vi "NI VeriStand - Start Multiple Waveforms Multi t0 (DBL).vi"(8 "error in (no error)":errorcluster, 10 "t0s":timestamp[](array[timestamp]), 11 "Multiple Waveforms Write Session (DBL) in":refnum<class "Multiple Waveforms Write (DBL).lvclass">) -> (0 "error out":errorcluster, 3 "Multiple Waveforms Write Session (DBL) out":refnum<class "Multiple Waveforms Write (DBL).lvclass">)   [LabVIEW 2020, in "NI_VS Custom Device Waveform API.lvlib" / "Multiple Waveforms Write (DBL).lvclass"]
doc: "Sets the start time (t0) for the waveform data you want to write with the Write Waveform(s) VI. NI VeriStand considers all data the custom device writes to a waveform be continuous unless this VI executes again with a different start time."
uses:
  Multiple Waveforms Write (DBL).lvclass
  D:/p4/penguin/lvaddon/Veristand/master/src/LabVIEW/vilib/NI VeriStand/Custom Device Waveform API/Waveform Session.lvclass
  Waveform Session.lvclass/Waveform Session.ctl
  Multiple Waveforms Write (DBL).lvclass/Multiple Waveforms Write (DBL).ctl
  Internal Comm Classes/WPL Comm/WPL Comm.lvclass/WPL Comm.ctl
  Internal Comm Classes/WPL Comm/Send WPL Command.vi
  Internal Comm Classes/WPL Comm/Set Multi t0 on Variant.vi
  Internal Comm Classes/WPL Comm/Convert Q Error to Shutdown Error.vi
  Internal Comm Classes/WPL Comm/WPL Comm (2D DBL)/WPL Comm (2D DBL).lvclass
  D:/p4/penguin/lvaddon/Veristand/master/src/LabVIEW/vilib/NI VeriStand/Custom Device Waveform API/Internal Comm Classes/WPL Comm/WPL Comm.lvclass
  <vilib>/Utility/error.llb/Error Cluster From Error Code.vi
  Waveform Session.lvclass
  Internal Comm Classes/WPL Comm/WPL Comm.lvclass
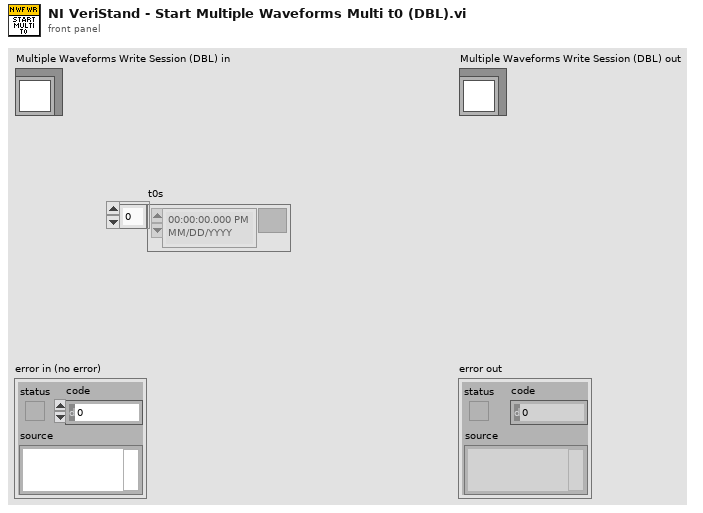
[diagram p1: front panel]
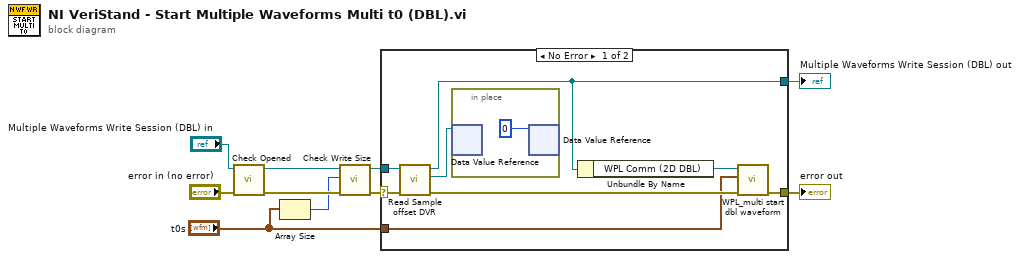
[diagram p0: block diagram]
diagram:
  n1 = call "Check Opened.vi"("error in (no error)"="error in (no error)", "Waveform Session in"="Multiple Waveforms Write Session (DBL) in") -> ("error out"=w3:errorcluster, "Waveform Session out"=w6:refnum<class "Multiple Waveforms Write (DBL).lvclass">)  [unwired: 8 in]
  n2 = Array Size(array="t0s") -> (size(s)=w1:i32)
  n3 = call "Check Write Size.vi"("error in (no error)"=w3, "# Of Waveforms"=w1, "Waveform Session in"=w6) -> ("error out"=w4:errorcluster, "Waveform Session out"=w5:refnum<class "Multiple Waveforms Write (DBL).lvclass">)  [unwired: 7 in]
  n4 = case shown="No Error" w4 {
    selector: w4 -> [w17 w20]
    tunnel: [w15 w20] -> w10
    tunnel: [w12 w19] -> w9
    tunnel: w5 -> [w13 w19]
    tunnel: "t0s" -> [w14 _]
    frame No Error {
      n5 = call "Read Sample offset DVR.vi"("Waveform Session in"=w13) -> ("Sample offset"=w11:refnum<data-value>, "Waveform Session out"=w12:refnum<class "Multiple Waveforms Write (DBL).lvclass">)  [unwired: 9 in]
      n6 = in-place {
        n7 = in-place-dvr #1(w11) -> ()  [unwired: 2 out]
        n8 = in-place-dvr #1(u64 0 ("data value")) -> ()  [unwired: 2 out]
      }
      n9 = Unbundle By Name(w12) -> ("WPL Comm (2D DBL)"=w16:refnum<class "WPL Comm (2D DBL).lvclass">)
      n10 = call "WPL_multi start dbl waveform.vi"("error in (no error)"=w17, "t0s"=w14, "WPL Comm in"=w16) -> ("error out"=w15:errorcluster)  [unwired: 8 in]
    }
    frame Error {
    }
  }
  "error out" <- w10
  "Multiple Waveforms Write Session (DBL) out" <- w9
